vi "CalcAngleChange.vi"(9 "Direction":dbl, 10 "Turret Angle":dbl, 11 "Linear speed":dbl) -> (3 "Angle Change":dbl)   [LabVIEW 2014]
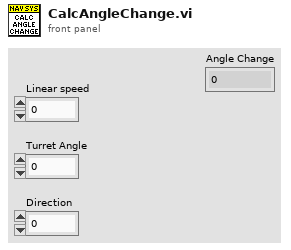
[diagram p1: front panel]
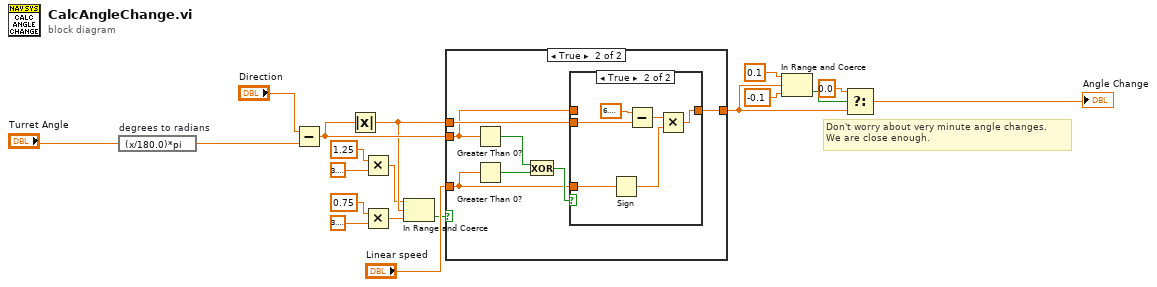
[diagram p0: block diagram]
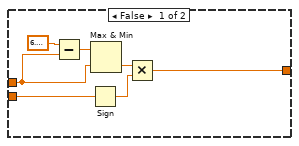
[diagram p2: hidden frame]
diagram:
  # "Don't worry about very minute angle changes.\nWe are close enough."
  n1 = expression code="(x/180.0)*pi" "degrees to radians"("Turret Angle") -> (w1:dbl)
  n2 = Subtract(x="Direction", y=w1) -> (x-y=w19:dbl)
  n3 = Absolute Value(x=w19) -> (abs(x)=w17:dbl)
  n4 = Multiply(x=1.25, y=3.141592653589793) -> (x*y=w15:dbl)
  n5 = Multiply(x=0.75, y=3.141592653589793) -> (x*y=w12:dbl)
  n6 = In Range and Coerce(upper limit=w15, x=w17, lower limit=w12) -> (In Range?=w16:bool)  [unwired: 1 out]
  n7 = case shown="True" w16 {
    tunnel: w17 -> [w24 w30]
    tunnel: [w22 w28] -> w4
    tunnel: "Linear speed" -> [_ w27]
    tunnel: w19 -> [w20 w29]
    frame False {
      n8 = Subtract(x=6.283185307179586, y=w24) -> (x-y=w25:dbl)
      n9 = Sign(1:w20) -> (0:w21:dbl)
      n10 = Max & Min(x=w25, y=w24) -> (min(x,y)=w23:dbl)  [unwired: 1 out]
      n11 = Multiply(x=w23, y=w21) -> (x*y=w22:dbl)
    }
    frame True {
      n12 = Greater Than 0?(x=w29) -> (x > 0?=w32:bool)
      n13 = Greater Than 0?(x=w27) -> (x > 0?=w33:bool)
      n14 = Exclusive Or(1:w33, 2:w32) -> (0:w31:bool)
      n15 = case shown="True" w31 {
        tunnel: w30 -> [_ w40]
        tunnel: w29 -> [w34 _]
        tunnel: [w34 w36] -> w28
        tunnel: w27 -> [_ w35]
        frame False {
        }
        frame True {
          n16 = Sign(1:w35) -> (0:w38:dbl)
          n17 = Subtract(x=6.283185307179586, y=w40) -> (x-y=w37:dbl)
          n18 = Multiply(x=w37, y=w38) -> (x*y=w36:dbl)
        }
      }
    }
  }
  n19 = In Range and Coerce(upper limit=0.1, x=w4, lower limit=-0.1) -> (In Range?=w6:bool)  [unwired: 1 out]
  n20 = Select(t=0.0, s=w6, f=w4) -> (s? t:f=→"Angle Change":dbl)
